vi "Real-Time LED_Turn Off.vi"(11 "error in (no error)":errorcluster) -> (14 "Roundtrip Time":dbl format="%.6fsec", 15 "error out":errorcluster)   [LabVIEW 2015]
uses:
  Real-Time LED_Color.ctl
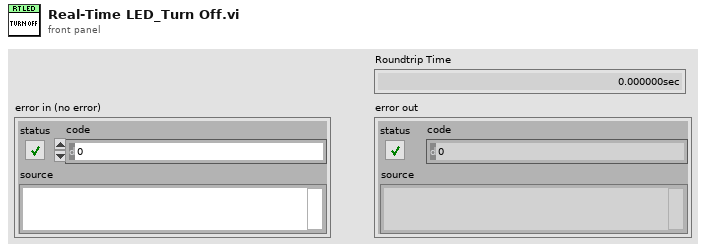
[diagram p1: front panel]
types:
  T1 = typedef "Real-Time LED_Color.ctl" = enum8{"Off", "Green", "Amber"}
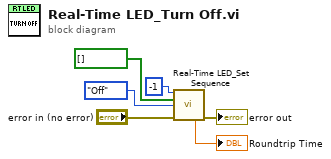
[diagram p0: block diagram]
diagram:
  n1 = call "Real-Time LED_Set Sequence.vi"("Flash Period"=-1, "Sequence"=bool[] [], "Color"=Real-Time_LED_Color."Off", "error in (no error)"="error in (no error)") -> ("Roundtrip Time"=→"Roundtrip Time":dbl, "error out"=→"error out":errorcluster)  [unwired: 10 in]
